vi "CS-4 Set Sweep Mode.vi"(4 "error in (no error)":errorcluster, 6 "sweep mode":T1, 7 "VISA session":refnum<visa-resource-name>) -> (0 "error out":errorcluster, 3 "dup VISA session":refnum<visa-resource-name>)   [LabVIEW 2016]
doc: "CS-4 Read Current.vi will return the present supply output current reading."
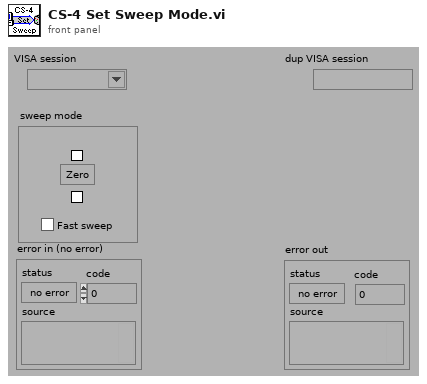
[diagram p1: front panel]
types:
  T1 = cluster{"zero":bool, "sweep up":bool, "sweep down":bool, "fast sweep":bool}
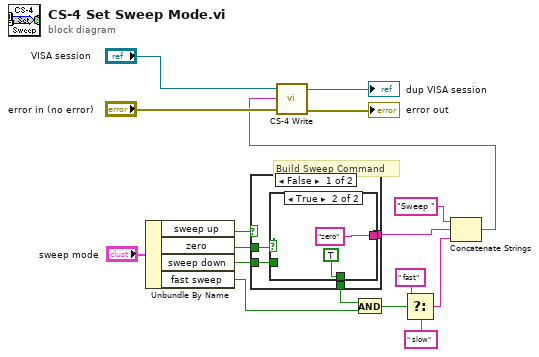
[diagram p0: block diagram]
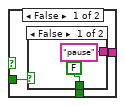
[diagram p2: hidden frame]
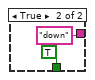
[diagram p3: hidden frame]
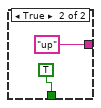
[diagram p4: hidden frame]
diagram:
  # "Build Sweep Command"
  n1 = Unbundle By Name("sweep mode") -> ("sweep up"=w14:bool, "zero"=w13:bool, "sweep down"=w12:bool, "fast sweep"=w10:bool)
  n2 = case shown="False" w14 {
    tunnel: [w20 "up"] -> w5
    tunnel: w13 -> [w21 _]
    tunnel: w12 -> [w19 _]
    tunnel: [w18 TRUE] -> w11
    frame False {
      n3 = case shown="True" w21 {
        tunnel: [w24 "zero"] -> w20
        tunnel: w19 -> [w22 _]
        tunnel: [w23 TRUE] -> w18
        frame False {
          n4 = case shown="False" w22 {
            tunnel: ["pause" "down"] -> w24
            tunnel: [FALSE TRUE] -> w23
            frame False {
            }
            frame True {
            }
          }
        }
        frame True {
        }
      }
    }
    frame True {
    }
  }
  n5 = And(x=w11, y=w10) -> (x .and. y?=w9:bool)
  n6 = Select(t=" fast", s=w9, f=" slow") -> (s? t:f=w4:string)
  n7 = Concatenate Strings("Sweep ", w5, w4) -> (w3:string)
  n8 = call "CS-4 Write.vi"("error in (no error)"="error in (no error)", "write buffer (\"\")"=w3, "VISA session"="VISA session") -> ("error out"=→"error out":errorcluster, "dup VISA session"=→"dup VISA session":refnum<visa-resource-name>)  [unwired: 1 out]
